vi "Write htx.vi"(8 "error in (no error)":errorcluster, 10 "htx":dbl, 11 "Update TE Tech Heating Params in":refnum<class "Update TE Tech Heating Params.lvclass">) -> (0 "error out":errorcluster, 3 "Update TE Tech Heating Params out":refnum<class "Update TE Tech Heating Params.lvclass">)   [LabVIEW 2014, in "Controller.lvlib" / "Update TE Tech Heating Params.lvclass"]
uses:
  Update TE Tech Heating Params.lvclass
  Update TE Tech Heating Params.lvclass/Update TE Tech Heating Params.ctl
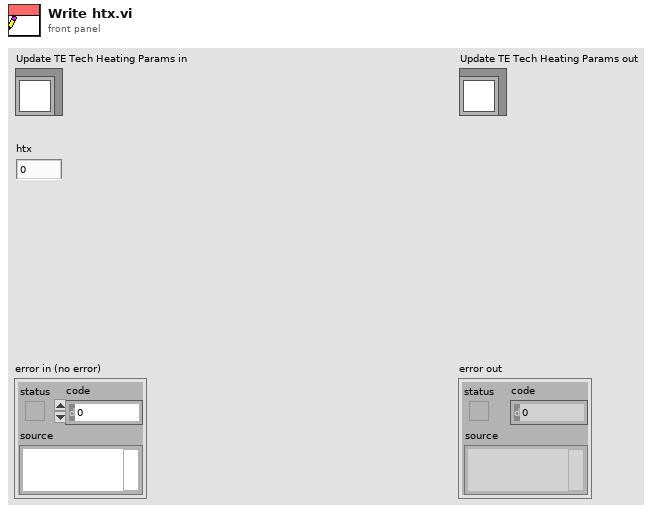
[diagram p1: front panel]
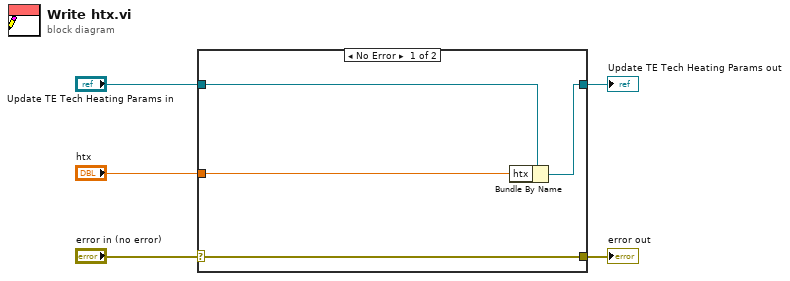
[diagram p0: block diagram]
diagram:
  n1 = case shown="No Error" "error in (no error)" {
    selector: "error in (no error)" -> [w9 w10]
    tunnel: [w9 w10] -> w4
    tunnel: [w7 w11] -> w2
    tunnel: "Update TE Tech Heating Params in" -> [w8 w11]
    tunnel: "htx" -> [w6 _]
    frame No Error {
      n2 = Bundle By Name(cluster=w8, "htx"=w6) -> (w7:refnum<class "Update TE Tech Heating Params.lvclass">)
    }
    frame Error {
    }
  }
  "error out" <- w4
  "Update TE Tech Heating Params out" <- w2
